vi "GetInterfacesInProject.vi"(8 "error in":errorcluster, 11 "Project/ProjectItem":variant) -> (0 "error out":errorcluster, 2 "InterfaceInfo":T1[](array[typedef]))   [LabVIEW 2020, in "InterfaceLibrary.lvlib"]
uses:
  <resource>/Framework/Providers/Open_GDS/ClassProviders/Common/InterfaceLibrary/InterfaceLibrary.lvlib
  <resource>/Framework/Providers/Open_GDS/ClassProviders/Common/InterfaceLibrary/InterfaceInfo.ctl
  <resource>/Framework/Providers/Open_GDS/ClassProviders/Common/LvClass_class/GDSLvClass_ClassMethodInfo.ctl
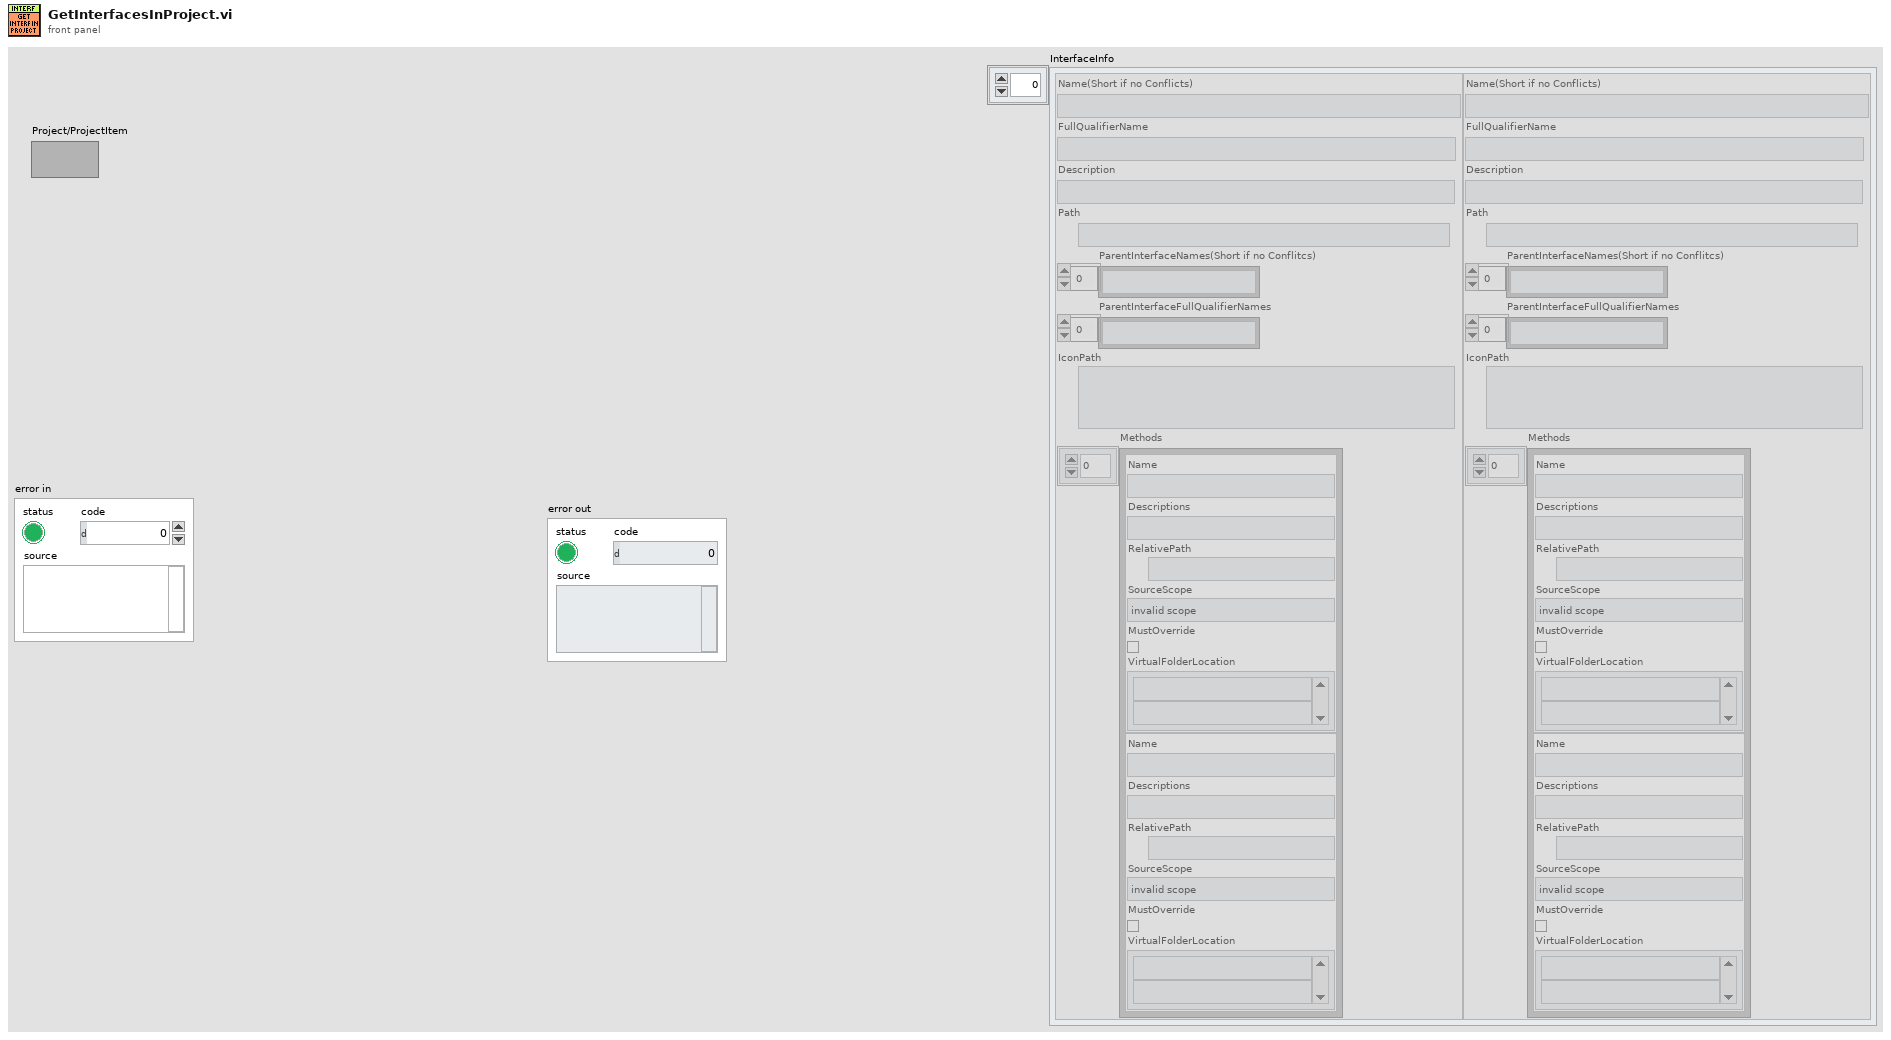
[diagram p1: front panel]
types:
  T1 = typedef "InterfaceLibrary.lvlib/InterfaceInfo.ctl" = cluster{"Name(Short if no Conflicts)":string, "FullQualifierName":string, "Description":string, "Path":path, "ParentInterfaceNames(Short if no Conflitcs)":string[], "ParentInterfaceFullQualifierNames":string[], "IconPath":path, "Methods":T2[]}
  T2 = typedef "GDSLvClass_ClassMethodInfo.ctl" = cluster{"Name":string, "Descriptions":string, "RelativePath":path, "SourceScope":enum32{"invalid scope", "public", "private", "protected", "community"}, "MustOverride":bool, "VirtualFolderLocation":string[]}
  T3 = enum32{"invalid scope", "public", "private", "protected", "community"}
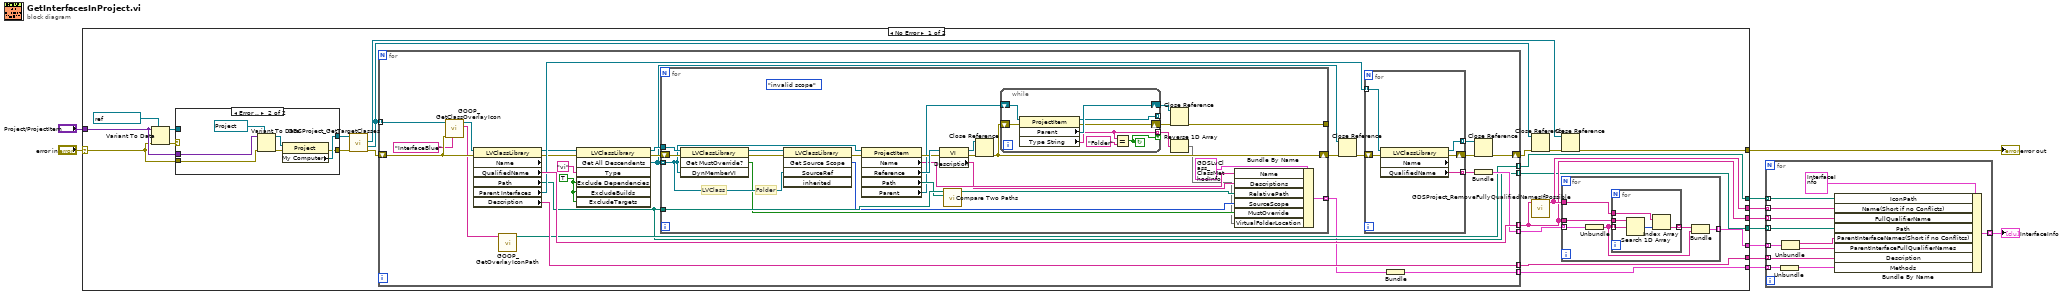
[diagram p0: block diagram]
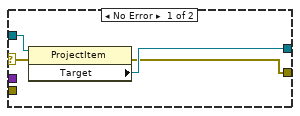
[diagram p2: hidden frame]
diagram:
  n1 = case shown="No Error" "error in" {
    selector: "error in" -> [w28 w120]
    tunnel: "Project/ProjectItem" -> [w29 _]
    tunnel: [w14 w120] -> w9
    tunnel: [w22 _] -> w7
    tunnel: [w21 _] -> w4
    tunnel: [w20 _] -> w6
    tunnel: [w19 _] -> w5
    tunnel: [w18 _] -> w3
    tunnel: [w17 _] -> w8
    tunnel: [w12 _] -> w1
    frame No Error {
      n2 = Variant To Data(error in=w28, type=refnum<vi> refnum ("ProjectItem"), Variant=w29) -> (data=w31:refnum<vi>, error out=w30:errorcluster)
      n3 = case shown="Error .." w30 {
        selector: w30 -> [w109 _]
        tunnel: w31 -> [w112 _]
        tunnel: [w111 w114] -> w27
        tunnel: [w110 w113] -> w26
        tunnel: w29 -> [_ w118]
        tunnel: w28 -> [_ w117]
        frame No Error {
          n4 = property class="ProjectItem"(reference=w112, error in=w109) -> (error out=w110:errorcluster, "Target"=w111:refnum<vi>)  [unwired: 1 out]
        }
        frame Error {
          n5 = Variant To Data(error in=w117, type=refnum<vi> refnum ("ProjectItem"), Variant=w118) -> (data=w116:refnum<vi>, error out=w115:errorcluster)
          n6 = property class="Project"(reference=w116, error in=w115) -> (error out=w113:errorcluster, "My Computer"=w114:refnum<vi>)  [unwired: 1 out]
        }
      }
      n7 = call <resource>:"GDSProject_GetTargetClasses.vi"("error in (no error)"=w26, "TargetItem in"=w27) -> ("error out"=w25:errorcluster, "LvInterfaces"=w16:refnum<vi>[], "LvClasses"=w13:refnum<vi>[])  [unwired: 6 in, 1 out]
      n8 = for {
        tunnel: w16 -> [w64] mode=indexing
        tunnel: [w69] -> w20 mode=indexing
        shift-right: [w51] -> w24
        shift-left: w25 -> [w62]
        tunnel: [w66] -> w23 mode=indexing
        tunnel: [w46] -> w19 mode=indexing
        tunnel: [w65] -> w18 mode=indexing
        tunnel: [w60] -> w17 mode=indexing
        tunnel: [w45] -> w12 mode=indexing
        w55 = TRUE ("ExcludeDependencies")
        n9 = call <resource>:"GOOP_GetClassOverlayIcon.vi"("DefaultIconName(BlueFull)"="InterfaceBlue", "error in (no error)"=w62, "LVClassLibrary in"=w64) -> ("IconName"=w61:string, "LVClassLibrary out"=w63:refnum<vi>)  [unwired: 6 in, 1 out]
        n10 = property class="LVClassLibrary" props=["Name", "QualifiedName", "Path", "Parent Interfaces", "Description"](reference=w63, error in=w62) -> (reference out=w56:refnum<vi>, error out=w57:errorcluster, "QualifiedName"=w69:string, "Path"=w46:path, "Parent Interfaces"=w68:refnum<vi>[], "Description"=w65:string)  [unwired: 1 out]
        n11 = call <resource>:"GOOP_GetOverlayIconPath.vi"("IconName(NoPngExtension)"=w61) -> ("IconPath"=w60:path)  [unwired: 10 in]
        n12 = invoke class="LVClassLibrary" method="Get All Descendents"(reference=w56, error in=w57, "Type"="vi", "Exclude Dependencies"=w55, "ExcludeBuilds"=w55, "ExcludeTargets"=w55) -> (reference out=w50:refnum<vi>, error out=w53:errorcluster, "All Descendents"=w47:refnum<vi>[])  [unwired: 1 in, 4 out]
        n13 = for {
          tunnel: w47 -> [w84] mode=indexing
          shift-right: [w80] -> w49
          shift-left: w53 -> [w90]
          tunnel: w50 -> [w91]
          tunnel: w46 -> [w89]
          tunnel: [w78] -> _
          tunnel: [w70] -> w44 mode=indexing
          (unwired) T3."invalid scope" ("Source Scope:Get")
          # "Folder"
          # "LVClass"
          n14 = invoke class="LVClassLibrary" method="Get MustOverride?"(reference=w91, error in=w90, "DynMemberVI"=w84) -> (reference out=w85:refnum<vi>, error out=w83:errorcluster, "GetMustOverride"=w72:bool)  [unwired: 1 in, 1 out]
          n15 = invoke class="LVClassLibrary" method="Get Source Scope"(reference=w85, error in=w83, "SourceRef"=w84) -> (error out=w82:errorcluster, "GetSourceScope"=w73:T3)  [unwired: 2 in, 3 out]
          n16 = property class="ProjectItem"(reference=w84, error in=w82) -> (error out=w93:errorcluster, "Name"=w76:string, "Reference"=w95:refnum<vi>, "Path"=w88:path, "Parent"=w87:refnum<vi>)  [unwired: 1 out]
          n17 = property class="VI"(reference=w95, error in=w93) -> (reference out=w94:refnum<vi>, error out=w92:errorcluster, "Description"=w75:string)
          n18 = call <vilib>:"Compare Two Paths.vi"("Path 2"=w88, "Path 1"=w89) -> ("Relative Path from 1 to 2"=w74:path)  [unwired: 6 in, 3 out]
          n19 = Close Reference(reference=w94, error in (no error)=w92) -> (error out=w80:errorcluster)
          n20 = while {
            tunnel: [w101] -> w86 mode=indexing if=w99
            shift-right: [w102] -> w81
            shift-left: w87 -> [w103]
            tunnel: [w98] -> _ mode=indexing
            shift-right: [w96] -> w79
            shift-left: w80 -> [w97]
            stop <- w99 continue-if-true
            n21 = property class="ProjectItem"(reference=w103, error in=w97) -> (reference out=w98:refnum<vi>, error out=w96:errorcluster, "Parent"=w102:refnum<vi>, "Type String"=w101:string)
            n22 = Equal?(x=w101, y="Folder") -> (x = y?=w99:bool)
          }
          n23 = Close Reference(reference=w81, error in (no error)=w79) -> (error out=w78:errorcluster)
          n24 = Reverse 1D Array(array=w86) -> (reversed array=w71:string[])
          n25 = Bundle By Name(cluster=T2 {"Name"="", "Descriptions"="", "RelativePath"=path "", "SourceScope"=enum."invalid scope", "MustOverride"=FALSE, "VirtualFolderLocation"=[]} ("MethodSettings"), "Name"=w76, "Descriptions"=w75, "RelativePath"=w74, "SourceScope"=w73, "MustOverride"=w72, "VirtualFolderLocation"=w71) -> (w70:T2)
        }
        n26 = Close Reference(reference=w47, error in (no error)=w49) -> (error out=w48:errorcluster)
        n27 = for {
          tunnel: w68 -> [w108] mode=indexing
          tunnel: [w107] -> w67 mode=indexing
          tunnel: [w106] -> w58 mode=indexing
          shift-right: [w104] -> w52
          shift-left: w48 -> [w105]
          n28 = property class="LVClassLibrary" props=["Name", "QualifiedName"](reference=w108, error in=w105) -> (reference out=w106:refnum<vi>, error out=w104:errorcluster, "QualifiedName"=w107:string)  [unwired: 1 out]
        }
        n29 = Bundle(w44) -> (w45:cluster{T2[]})  [unwired: 1 in]
        n30 = Close Reference(reference=w58, error in (no error)=w52) -> (error out=w51:errorcluster)
        n31 = Bundle(w67) -> (w66:cluster{string[]})  [unwired: 1 in]
      }
      n32 = Close Reference(reference=w16, error in (no error)=w24) -> (error out=w15:errorcluster)
      n33 = call <resource>:"GDSProject_RemoveFullyQualifiedNamesIfPossible.vi"("ItemnamesIn"=w20) -> ("ItemnamesOut"=w22:string[])  [unwired: 10 in]
      n34 = Close Reference(reference=w13, error in (no error)=w15) -> (error out=w14:errorcluster)
      n35 = for {
        tunnel: w23 -> [w38] mode=indexing
        tunnel: w20 -> [w37]
        tunnel: w22 -> [w36]
        tunnel: [w34] -> w21 mode=indexing
        n36 = Unbundle(w38) -> (w33:string[])
        n37 = for {
          tunnel: w33 -> [w43] mode=indexing
          tunnel: w37 -> [w42]
          tunnel: w36 -> [w40]
          tunnel: [w39] -> w35 mode=indexing
          n38 = Search 1D Array(1D array=w42, element=w43) -> (index of element=w41:i32)  [unwired: 1 in]
          n39 = Index Array(array=w40, index=w41) -> (element=w39:string)
        }
        n40 = Bundle(w35, w33) -> (w34:cluster{string[], string[]})  [unwired: 1 in]
      }
    }
    frame Error {
    }
  }
  "error out" <- w9
  n41 = for {
    tunnel: w8 -> [w132] mode=indexing
    tunnel: w7 -> [w131] mode=indexing
    tunnel: w6 -> [w130] mode=indexing
    tunnel: w5 -> [w129] mode=indexing
    tunnel: w4 -> [w128] mode=indexing
    tunnel: w3 -> [w125] mode=indexing
    tunnel: [w123] -> w2 mode=indexing
    tunnel: w1 -> [w122] mode=indexing
    n42 = Unbundle(w122) -> (w121:T2[])
    n43 = Unbundle(w128) -> (w127:string[], w126:string[])
    n44 = Bundle By Name(cluster=T1 {"Name(Short if no Conflicts)"="", "FullQualifierName"="", "Description"="", "Path"=path "", "ParentInterfaceNames(Short if no Conflitcs)"=[], "ParentInterfaceFullQualifierNames"=[], "IconPath"=path "", "Methods"=[]} ("InterfaceInfo"), "IconPath"=w132, "Name(Short if no Conflicts)"=w131, "FullQualifierName"=w130, "Path"=w129, "ParentInterfaceNames(Short if no Conflitcs)"=w127, "ParentInterfaceFullQualifierNames"=w126, "Description"=w125, "Methods"=w121) -> (w123:T1)
  }
  "InterfaceInfo" <- w2
